vi "UI_Center FP.vi"(8 "Error":errorcluster, 11 "VI Ref":refnum<vi>) -> (0 "Error Out":errorcluster, 3 "VI Ref Out":refnum<vi>)   [LabVIEW 2009]
doc: "Centers the VI's Front Panel to the Primary Monitor."
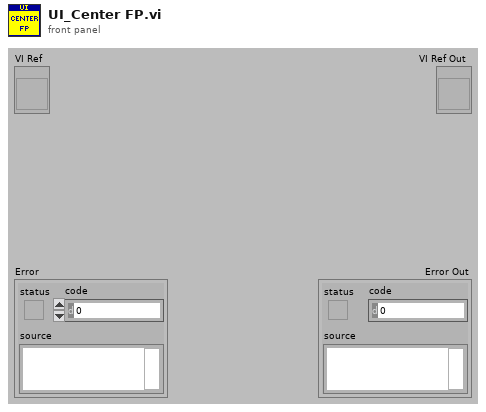
[diagram p1: front panel]
types:
  T1 = typedef "LVRectTypeDef.ctl" = cluster{"left":i16, "top":i16, "right":i16, "bottom":i16}
  T2 = cluster{"left":i16, "top":i16, "right":i16, "bottom":i16}
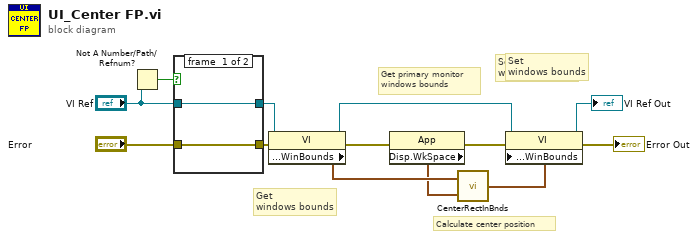
[diagram p0: block diagram]
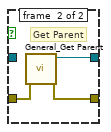
[diagram p2: hidden frame]
diagram:
  # "Get\nwindows bounds"
  # "Set\nwindows bounds"
  # "Set\nwindows bounds"
  # "Get primary monitor \nwindows bounds"
  # "Calculate center position"
  n1 = Not A Number/Path/Refnum?(number/path/refnum="VI Ref") -> (NaN/Path/Refnum?=w4:bool)
  n2 = case shown="True" w4 {
    tunnel: [w15 w18] -> w5
    tunnel: "VI Ref" -> [w15 _]
    tunnel: "Error" -> [w14 w17]
    tunnel: [w14 w16] -> w1
    frame #0 {
    }
    frame #1 {
      # "Get Parent"
      n3 = call "General_Get Parent.vi"("Error In (no Error)"=w17) -> ("Error Out"=w16:errorcluster, "VI Refnum Out"=w18:refnum<vi>)  [unwired: 8 in, 1 out]
    }
  }
  n4 = property class="VI"(reference=w5, error in=w1) -> (reference out=w11:refnum<vi>, error out=w10:errorcluster, "Front Panel.WinBounds"=w13:T1)
  n5 = property class="App"(error in=w10) -> (error out=w9:errorcluster, "Disp.WkSpace"=w12:T1)  [unwired: 1 in, 1 out]
  n6 = call <vilib>:"CenterRectInBnds.vi"("bounds"=w12, "rect"=w13) -> ("centered rect"=w6:T2)
  n7 = property class="VI"(reference=w11, error in=w9, "Front Panel.WinBounds"=w6) -> (reference out=→"VI Ref Out":refnum<vi>, error out=→"Error Out":errorcluster)
